vi "ConnectionListener.vi"(0 "reference in":refnum<class "Websocket.lvclass">, 5 "error in":errorcluster) -> (14 "reference out":refnum<class "Websocket.lvclass">, 19 "error out":errorcluster)   [LabVIEW 2014, in "FrontPanelPublisher.lvlib" / "Websocket.lvclass"]
uses:
  Websocket.lvclass
  Common/SHA-1.vi
  Common/Convert to Base64.vi
  Common/SHA-1 Digest.vi
  Common/SHA-1 Core.vi
  Common/SHA-1 Pad.vi
  <vilib>/Utility/error.llb/Trim Whitespace.vi
panel:
  out "Stop":bool
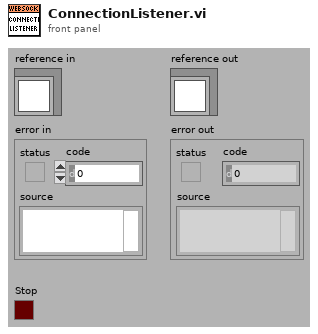
[diagram p1: front panel]
types:
  T1 = typedef "FrontPanelPublisher.lvlib/Websocket.lvclass/ObjectAttributes.ctl" = cluster{"Port":u16, "TCP Refs":refnum<k5>[], "Connection IDs":u64[]}
  T2 = enum16{"Standard", "Buffered", "CRLF", "Immediate"}
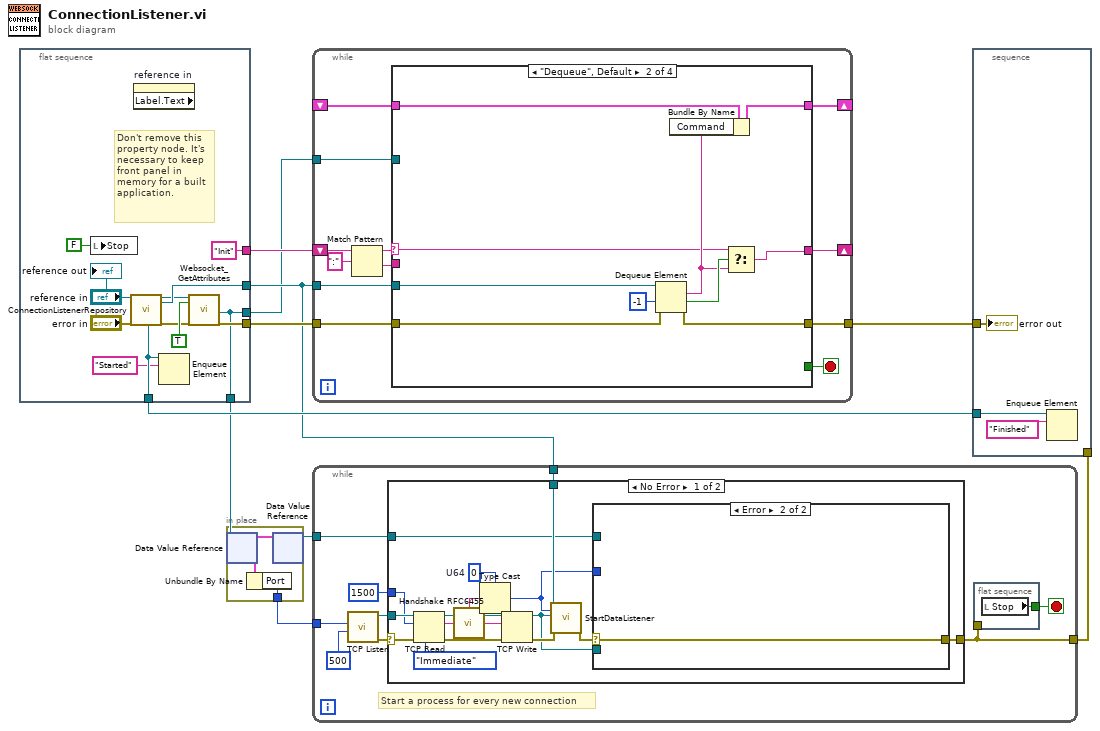
[diagram p0: block diagram]
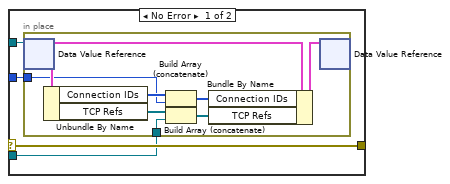
[diagram p2: hidden frame]
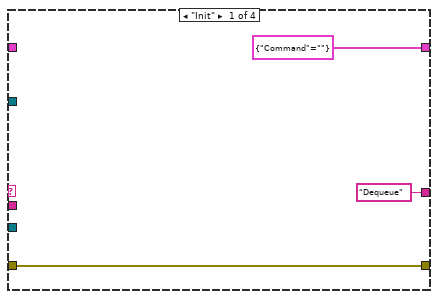
[diagram p4: hidden frame]
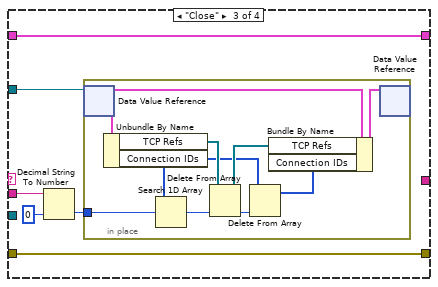
[diagram p5: hidden frame]
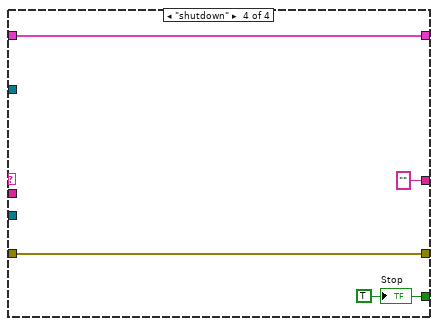
[diagram p6: hidden frame]
diagram:
  n1 = flat-sequence {
    tunnel: [w13] -> w10
    tunnel: [w22] -> w3
    tunnel: [w21] -> w8
    tunnel: ["Init"] -> w7
    tunnel: [w12] -> w5
    tunnel: [w12] -> w2
    frame #0 {
      # "Don't remove this property node. It's necessary to keep front panel in memory for a built application."
      n2 = local write "Stop"(FALSE ("Stop")) -> ()
      n3 = call "ConnectionListenerRepository.vi"("reference in"="reference in", "error in (no error)"="error in") -> ("ProcessSyncQueue"=w21:refnum<queue>, "reference out"=w15:refnum<class "Websocket.lvclass">, "ToProcessQueue"=w22:refnum<queue>, "error out"=w14:errorcluster)  [unwired: 11 in, 3 out]
      n4 = property on="reference in" class="LVClassControl (strict)" props=["Label", "Text"]() -> ()  [unwired: 2 in, 3 out]
      n5 = Enqueue Element(queue=w21, element="Started") -> ()  [unwired: 2 in, 3 out]
      n6 = call "Websocket_GetAttributes.vi"("reference in"=w15, "OnlyGetDvrReference(False)"=TRUE, "error in (no error)"=w14) -> ("DataRef"=w12:refnum<data-value>, "error out"=w13:errorcluster)  [unwired: 13 in, 2 out]
      "reference out" <- "reference in"
    }
  }
  n7 = in-place {
    in-place-border: [w23] -> w6
    n8 = in-place-dvr #1(w5) -> (w24:T1)  [unwired: 1 out]
    n9 = Unbundle By Name(w24) -> ("Port"=w23:u16)
    n10 = in-place-dvr #1(w24) -> (w1:refnum<data-value>)  [unwired: 1 out]
  }
  n11 = while {
    tunnel: w3 -> [w35]
    shift-right: [w26] -> _
    shift-left: w7 -> [w33]
    shift-right: [w30] -> _
    shift-left: _ -> [w29]
    tunnel: w10 -> [w27]
    tunnel: [w36] -> w9
    tunnel: w2 -> [w25]
    stop <- w28 stop-if-true
    n12 = Match Pattern(string=w33, regular expression=":") -> (before substring=w32:string, after substring=w31:string)  [unwired: 1 in, 2 out]
    n13 = case shown="\"Dequeue\", Default" w32 {
      selector: w32 -> [_ w40 _ _]
      tunnel: w27 -> [w38 w49 w53 w67]
      tunnel: [w38 w48 w53 w67] -> w36
      tunnel: w35 -> [_ w46 _ _]
      tunnel: w31 -> [_ _ w55 _]
      tunnel: ["Dequeue" ("t") w44 _ "" ("y")] -> w26
      tunnel: [cluster{"Command":string} {"Command"=""} ("LocalVariable") w41 w52 w65] -> w30
      tunnel: w29 -> [_ w42 w52 w65]
      tunnel: [_ _ _ w64] -> w28
      tunnel: w25 -> [_ _ w51 _]
      frame "Init" {
      }
      frame "Dequeue", Default {
        n14 = Dequeue Element(queue=w46, timeout in ms (-1)=-1, error in (no error)=w49) -> (element=w43:string, timed out?=w45:bool, error out=w48:errorcluster)  [unwired: 1 out]
        n15 = Bundle By Name(cluster=w42, "Command"=w43) -> (w41:cluster{"Command":string})
        n16 = Select(t=w40, s=w45, f=w43) -> (s? t:f=w44:string)
      }
      frame "Close" {
        n17 = Decimal String To Number(string=w55, default (0L)=u64 0 ("default (0 I32)")) -> (number=w50:u64)  [unwired: 1 in, 1 out]
        n18 = in-place {
          in-place-border: w50 -> [w61]
          n19 = in-place-dvr #2(w51) -> (w63:T1)  [unwired: 1 out]
          n20 = Unbundle By Name(w63) -> ("TCP Refs"=w60:refnum<k5>[], "Connection IDs"=w58:u64[])
          n21 = Search 1D Array(1D array=w58, element=w61) -> (index of element=w56:i32)  [unwired: 1 in]
          n22 = Delete From Array(array=w60, index=w56) -> (array with subset deleted=w59:refnum<k5>[])  [unwired: 1 in, 1 out]
          n23 = Delete From Array(array=w58, index=w56) -> (array with subset deleted=w57:u64[])  [unwired: 1 in, 1 out]
          n24 = Bundle By Name(cluster=w63, "TCP Refs"=w59, "Connection IDs"=w57) -> (w62:T1)
          n25 = in-place-dvr #2(w62) -> ()  [unwired: 2 out]
        }
      }
      frame "shutdown" {
        w64 = TRUE
        "Stop" <- w64
      }
    }
  }
  n26 = while {
    tunnel: w6 -> [w73]
    tunnel: [w69] -> w4
    tunnel: w3 -> [w71]
    tunnel: w1 -> [w68]
    stop <- w70 stop-if-true
    # "Start a process for every new connection"
    n27 = call <vilib>:"TCP Listen.vi"("timeout ms (wait forever: -1)"=500, "port"=w73) -> ("error out"=w75:errorcluster, "connection ID"=w76:refnum<k5>)  [unwired: 5 in, 3 out]
    n28 = case shown="No Error" w75 {
      selector: w75 -> [w94 w108]
      tunnel: w76 -> [w87 _]
      tunnel: [w80 w108] -> w69
      tunnel: 1500 ("timeout ms (wait forever: -1)") -> [w85 _]
      tunnel: w71 -> [w83 _]
      tunnel: w68 -> [w82 _]
      frame No Error {
        w91 = u64 0  # U64
        n29 = TCP Read(connection ID=w87, bytes to read=w85, error in (no error)=w94, 7:T2."Immediate" ("mode (standard)")) -> (connection ID out=w86:refnum<k5>, data out=w89:string, error out=w93:errorcluster)  [unwired: 1 in]
        n30 = call "Handshake RFC6455.vi"("websocket client handshake"=w89) -> ("accept string"=w90:string, "websocket server handshake"=w92:string)
        n31 = Type Cast(type=w91, x=w90) -> (*(type *) &x=w79:u64)
        n32 = TCP Write(connection ID=w86, data in=w92, error in (no error)=w93) -> (connection ID out=w78:refnum<k5>, error out=w84:errorcluster)  [unwired: 1 in, 1 out]
        n33 = call "StartDataListener.vi"("ConListenerQ"=w83, "Connection ID"=w79, "TCP  Ref"=w78, "error in (no error)"=w84) -> ("error out"=w81:errorcluster)  [unwired: 15 in]
        n34 = case shown="Error" w81 {
          selector: w81 -> [w97 w107]
          tunnel: w82 -> [w98 _]
          tunnel: [w97 w107] -> w80
          tunnel: w79 -> [w96 _]
          tunnel: w78 -> [w95 _]
          frame No Error {
            n35 = in-place {
              in-place-border: w96 -> [w100]
              in-place-border: w95 -> [w99]
              n36 = in-place-dvr #3(w98) -> (w106:T1)  [unwired: 1 out]
              n37 = Unbundle By Name(w106) -> ("Connection IDs"=w104:u64[], "TCP Refs"=w103:refnum<k5>[])
              n38 = Build Array (concatenate)(w104, w100) -> (w102:u64[])
              n39 = Build Array (concatenate)(w103, w99) -> (w101:refnum<k5>[])
              n40 = Bundle By Name(cluster=w106, "Connection IDs"=w102, "TCP Refs"=w101) -> (w105:T1)
              n41 = in-place-dvr #3(w105) -> ()  [unwired: 2 out]
            }
          }
          frame Error {
          }
        }
      }
      frame Error {
      }
    }
    n42 = flat-sequence {
      tunnel: [w77] -> w70
      tunnel: w69 -> [_]
      frame #0 {
        n43 = local read "Stop"() -> (w77:bool)
      }
    }
  }
  n44 = stacked-sequence {
    tunnel: w9 -> [w111]
    tunnel: w8 -> [w110]
    tunnel: w4 -> [_]
    frame #0 {
      n45 = Enqueue Element(queue=w110, element="Finished") -> ()  [unwired: 2 in, 3 out]
      "error out" <- w111
    }
  }
